vi "Processing.Run.vi"(8 "error in (no error)":errorcluster) -> (0 "error out":errorcluster)   [LabVIEW 2019, in "Tools.lvlib"]
uses:
  Tools.lvlib
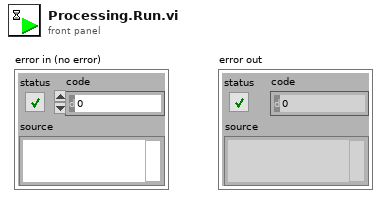
[diagram p1: front panel]
types:
  T1 = enum32{"Bad", "Idle", "Run top level", "Running"}
  T2 = enum32{"Invalid", "Standard", "Closed", "Hidden", "Minimized", "Maximized"}
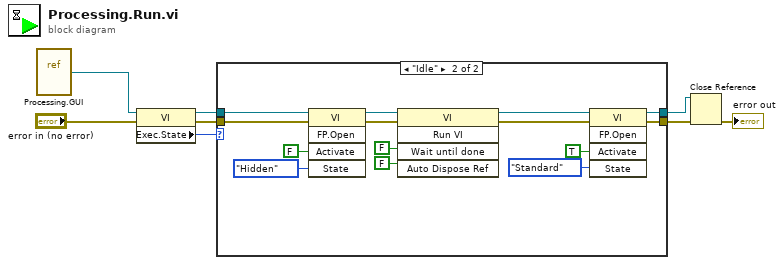
[diagram p0: block diagram]
diagram:
  n1 = vi-ref "Processing.GUI.vi"() -> (w3:refnum<vi>)
  n2 = property class="VI"(reference=w3, error in="error in (no error)") -> (reference out=w2:refnum<vi>, error out=w4:errorcluster, "Exec.State"=w1:T1)
  n3 = case shown="\"Idle\"" w1 {
    tunnel: [w9 w16] -> w6
    tunnel: [w10 w15] -> w5
    tunnel: w4 -> [w9 w12]
    tunnel: w2 -> [w10 w11]
    frame Default {
    }
    frame "Idle" {
      n4 = invoke class="VI" method="FP.Open"(reference=w11, error in=w12, "Activate"=FALSE ("Activate?"), "State"=T2."Hidden") -> (reference out=w22:refnum<vi>, error out=w19:errorcluster)  [unwired: 1 in, 3 out]
      n5 = invoke class="VI" method="Run VI"(reference=w22, error in=w19, "Wait until done"=FALSE ("Wait Until Done"), "Auto Dispose Ref"=FALSE ("Auto Dispose Reference")) -> (reference out=w18:refnum<vi>, error out=w17:errorcluster)  [unwired: 1 in, 3 out]
      n6 = invoke class="VI" method="FP.Open"(reference=w18, error in=w17, "Activate"=TRUE ("Activate?"), "State"=T2."Standard") -> (reference out=w15:refnum<vi>, error out=w16:errorcluster)  [unwired: 1 in, 3 out]
    }
  }
  n7 = Close Reference(reference=w5, error in (no error)=w6) -> (error out=→"error out":errorcluster)
